vi "SPI.vi"(0 "System no.":i32=1 min=1 max=4 step=1, 1 "Pivot point coordinates":cluster{"R":dbl, "S":dbl, "T":dbl} {"T" format="%.4f"; "S" format="%.4f"; "R" format="%.4f"}, 5 "error in":errorcluster) -> (14 "Controller error":bool, 19 "error out":errorcluster)   [LabVIEW 2020]
doc: "C-886, C-887, F-206- and M-8X0-specific. Sets the pivot point. Command will only be executed if all angular coordinates of current position are zero. Controller error is TRUE if selected system reports an error code which is not 0.\nCan only be used if a coordinate system of types KSF or ZERO is active.\n\nC-886, C-887, F-206, M-8X0: Pivot point coordinates (R,S,T) and (X,Y,Z) are valid and identical."
panel:
  # "Hexapod specific. Sets the Pivot Point. \nCommand will only be executed if all angular\ncoordinates of current position are zero."
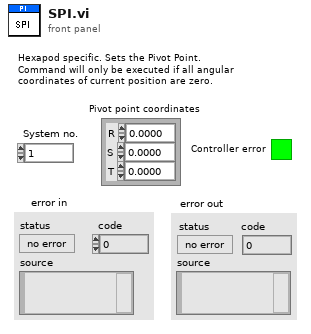
[diagram p1: front panel]
types:
  T1 = enum16{"Disable error check", "Force error check", "Use global settings"}
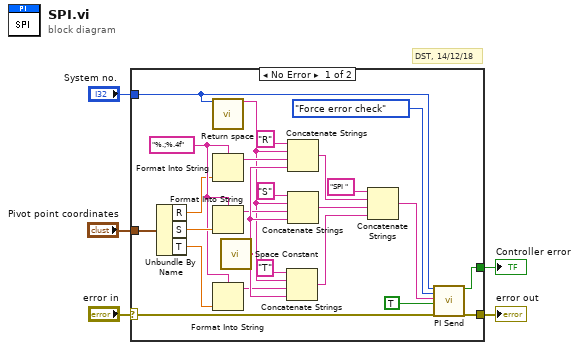
[diagram p0: block diagram]
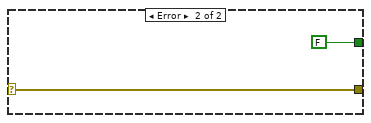
[diagram p2: hidden frame]
diagram:
  # "DST, 14/12/18"
  n1 = case shown="No Error" "error in" {
    selector: "error in" -> [w6 w31]
    tunnel: "Pivot point coordinates" -> [w25 _]
    tunnel: "System no." -> [w11 _]
    tunnel: [w8 FALSE ("Controller error")] -> w3
    tunnel: [w7 w31] -> w2
    frame No Error {
      w16 = "%.;%.4f" ("Format String")
      n2 = Unbundle By Name(w25) -> ("R"=w15:dbl, "S"=w18:dbl, "T"=w17:dbl)
      n3 = call "Return space.vi"("System no."=w11) -> ("String out"=w10:string)  [unwired: 1 in, 17 out]
      n4 = Format Into String(format string=w16, w15) -> (resulting string=w14:string)  [unwired: 2 in, 1 out]
      n5 = Format Into String(format string=w16, w18) -> (resulting string=w13:string)  [unwired: 2 in, 1 out]
      n6 = Format Into String(format string=w16, w17) -> (resulting string=w12:string)  [unwired: 2 in, 1 out]
      n7 = call "Space Constant.vi"() -> ("String"=w29:string)
      n8 = Concatenate Strings("T", w10, w12, w29) -> (w22:string)
      n9 = Concatenate Strings("R", w10, w14, w29) -> (w24:string)
      n10 = Concatenate Strings("S", w10, w13, w29) -> (w23:string)
      n11 = Concatenate Strings("SPI ", w24, w23, w22) -> (w19:string)
      n12 = call "PI Send.vi"("System no."=w11, "Error check settings"=T1."Force error check", "String to send"=w19, "Attach termination char.?"=TRUE ("Attach Linefeed?"), "error in"=w6) -> ("Controller error"=w8:bool, "error out"=w7:errorcluster)  [unwired: 1 in, 12 out]
    }
    frame Error {
    }
  }
  "error out" <- w2
  "Controller error" <- w3
